vi "Wojtek Controller.vi"(11 "Speed":dbl=0.5 format="%#_13g") -> ()   [LabVIEW 2013]
uses:
  Angle.vi
  <vilib>/Rock Robotics/WPI/RobotDrive/WPI_RobotDriveGetSetRefNum.vi
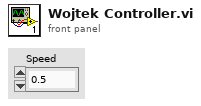
[diagram p1: front panel]
types:
  T1 = typedef "WPI_RobotDriveDevRef.ctl" = cluster{"DevStatus":errorcluster, "Motors[]":T2[], "Square Inputs":bool, "Max Output":dbl, "Isochronous":bool}
  T2 = typedef "WPI_MotorControlDeviceRef.ctl" = cluster{"DeviceStatus":errorcluster, "Type":enum16{"PWM", "CAN"}, "PWM":cluster{"Digital Module":T3, "PWM Channel":T4, "DeadBand":T5}, "CAN":cluster{"Device Number":u8, "Control Mode":T6, "Semaphore":T7, "Max Vout":dbl}, "Invert":bool, "TransformRef":T8, "InvTransformRef":T8}
  T3 = typedef "FPGA_TypedefDigitalModule.ctl" = enum16{"Digital Module 1", "Digital Module 2"}
  T4 = typedef "FPGA_DIOPWMChannel.ctl" = enum8{"PWM 1", "PWM 2", "PWM 3", "PWM 4", "PWM 5", "PWM 6", "PWM 7", "PWM 8", "PWM 9", "PWM 10", "Invalid"}
  T5 = typedef "WPI_PWMDeadband.ctl" = cluster{"Name":string, "maxPositivePwm":i32, "minPositivePwm":i32, "centerPwm":i32, "maxNegativePwm":i32, "minNegativePwm":i32, "angularRange":u16}
  T6 = typedef "WPI_CANJaguar_ControlMode.ctl" = enum8{"Percent VBus", "Current", "Speed", "Position", "Voltage"}
  T7 = typedef "Semaphore RefNum" = refnum<k1>
  T8 = typedef "WPI_PWMTransform_ConPane.ctl" = refnum<vi>
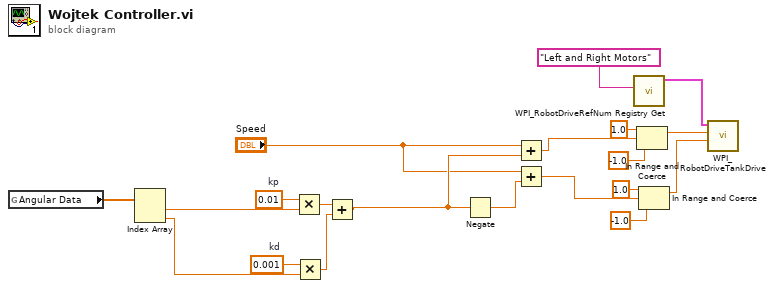
[diagram p0: block diagram]
diagram:
  w15 = 0.001  # kd
  w18 = 0.01  # kp
  n1 = global read "Angle.vi" "Angular Data"() -> (w16:dbl[])
  n2 = Index Array(array=w16) -> (element #1=w11:dbl, element #2=w10:dbl)  [unwired: 2 in]
  n3 = Multiply(x=w18, y=w11) -> (x*y=w17:dbl)
  n4 = Multiply(x=w15, y=w10) -> (x*y=w14:dbl)
  n5 = Add(x=w17, y=w14) -> (x+y=w8:dbl)
  n6 = Negate(x=w8) -> (-x=w9:dbl)
  n7 = Add(x="Speed", y=w8) -> (x+y=w2:dbl)
  n8 = Add(x="Speed", y=w9) -> (x+y=w7:dbl)
  n9 = call <vilib>:"WPI_RobotDriveRefNum Registry Get.vi"("refnum name"="Left and Right Motors") -> ("RobotDriveDevRef"=w20:T1)  [unwired: 1 in, 9 out]
  n10 = In Range and Coerce(upper limit=1.0, x=w2, lower limit=-1.0) -> (coerced(x)=w4:dbl)  [unwired: 1 out]
  n11 = In Range and Coerce(upper limit=1.0, x=w7, lower limit=-1.0) -> (coerced(x)=w3:dbl)  [unwired: 1 out]
  n12 = call <vilib>:"WPI_RobotDriveTankDrive.vi"("Right axis value"=w3, "Left axis value"=w4, "RobotDriveDevRef"=w20) -> ()  [unwired: 6 in, 3 out]
